vi "Disabled.vi"(7 "Robot Mode":T2, 10 "Match Info":T1={"Autonomous Elapsed Seconds"=0.0, "TeleOp Elapsed Seconds"=0.0, "Disabled Elapsed Seconds"=0.0, "Visited Autonomous"=FALSE, "Visited TeleOp"=FALSE, "Visited Disabled"=FALSE, "Autonomous Settings"={"Autonomous Style"=enum."Independent", "VI Refnum"=refnum}}, 11 "Call Context":T3) -> ()   [LabVIEW 2014]
doc: "This VI is called each time a disabled packet is received from the DS. It is often used to prepare for the next robot mode, to calibrate sensors, etc."
uses:
  <vilib>/Rock Robotics/WPI/DriverStation/WPI_DriverStationDerivedRobotMode.ctl
  <vilib>/Rock Robotics/WPI/DriverStation/WPI_DriverStationRobotMode2.ctl
  <vilib>/Rock Robotics/WPI/DriverStation/WPI_DriverStationMatch Info.ctl
  Robot Global Data.vi
panel:
  out "Numeric":dbl
  out "Pressed?":bool
  out "Voltage":dbl
  in  "Reset":bool
  out "Distance (in)":dbl
  out "Angle":dbl
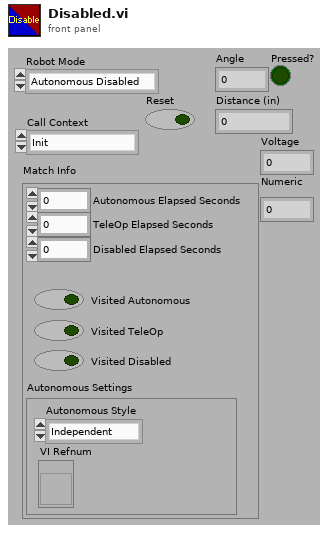
[diagram p1: front panel]
types:
  T1 = typedef "WPI_DriverStationMatch Info.ctl" = cluster{"Autonomous Elapsed Seconds":dbl, "TeleOp Elapsed Seconds":dbl, "Disabled Elapsed Seconds":dbl, "Visited Autonomous":bool, "Visited TeleOp":bool, "Visited Disabled":bool, "Autonomous Settings":cluster{"Autonomous Style":enum16{"Iterative", "Independent"}, "VI Refnum":refnum<vi>}}
  T2 = typedef "WPI_DriverStationRobotMode2.ctl" = enum16{"Autonomous Disabled", "Autonomous Enabled", "Teleop Disabled", "Teleop Enabled", "Disconnected", "Finish", "Test Disabled", "Test Enabled"}
  T3 = typedef "WPI_DriverStationDerivedRobotMode.ctl" = enum16{"Init", "Execute", "Stop"}
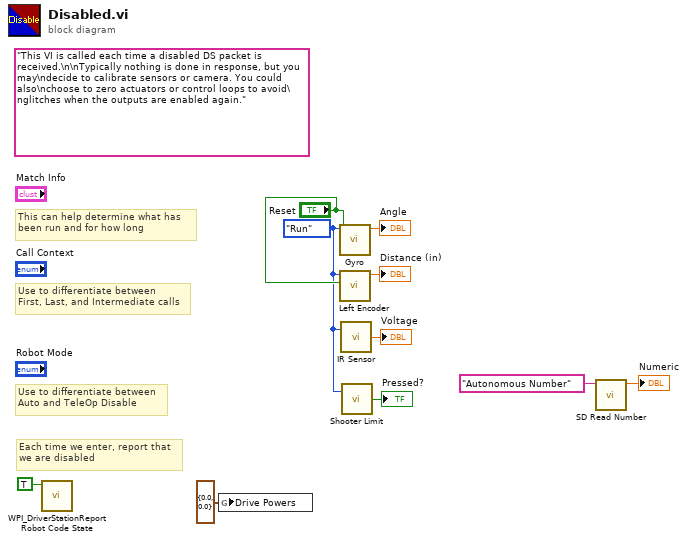
[diagram p0: block diagram]
diagram:
  w5 = enum16{"Start", "Run", "End"}."Run" ("Enum")
  (unwired) "This VI is called each time a disabled DS packet is received.\n\nTypically nothing is done in response, but you may\ndecide to calibrate sensors or camera. You could also\nchoose to zero actuators or control loops to avoid\nglitches when the outputs are enabled again."
  # "Each time we enter, report that\nwe are disabled"
  # "Use to differentiate between\nFirst, Last, and Intermediate calls"
  # "This can help determine what has\nbeen run and for how long"
  # "Use to differentiate between\nAuto and TeleOp Disable"
  n1 = call <vilib>:"WPI_DriverStationReport Robot Code State.vi"("Disabled"=TRUE ("Autonomous")) -> ()  [unwired: 10 in, 1 out]
  n2 = global write "Robot Global Data.vi" "Drive Powers"(cluster{"Right":dbl, "Left":dbl} {"Right"=0.0, "Left"=0.0} ("Drive Powers")) -> ()
  n3 = call "Gyro.vi"("Reset"="Reset", "Enum"=w5) -> ("Angle"=→"Angle":dbl)  [unwired: 9 in]
  n4 = call "Left Encoder.vi"("Reset"="Reset", "Enum"=w5) -> ("Distance (in)"=→"Distance (in)":dbl)  [unwired: 8 in, 1 out]
  n5 = call "IR Sensor.vi"("Enum"=w5) -> ("Voltage"=→"Voltage":dbl)  [unwired: 1 in]
  n6 = call "Shooter Limit.vi"("Enum"=w5) -> ("Value"=→"Pressed?":bool)  [unwired: 1 in]
  n7 = call <vilib>:"SD Read Number.vi"("Name"="Autonomous Number") -> ("Numeric"=→"Numeric":dbl)  [unwired: 8 in, 2 out]
